vi "Serialize as XML.vi"(8 "error in (no error)":errorcluster, 10 "Nesting Level":i32, 11 "Attribute in":refnum<class "Attribute.lvclass">) -> (0 "error out":errorcluster, 2 "XML Fragment":string, 3 "Attribute out":refnum<class "Attribute.lvclass">)   [LabVIEW 2026, in "VILab.lvlib" / "Attribute.lvclass"]
uses:
  Attribute.lvclass
  Attribute.lvclass/Attribute.ctl
  Data Item/Data Item.lvclass
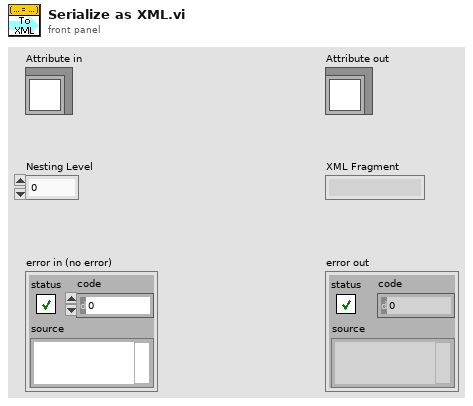
[diagram p1: front panel]
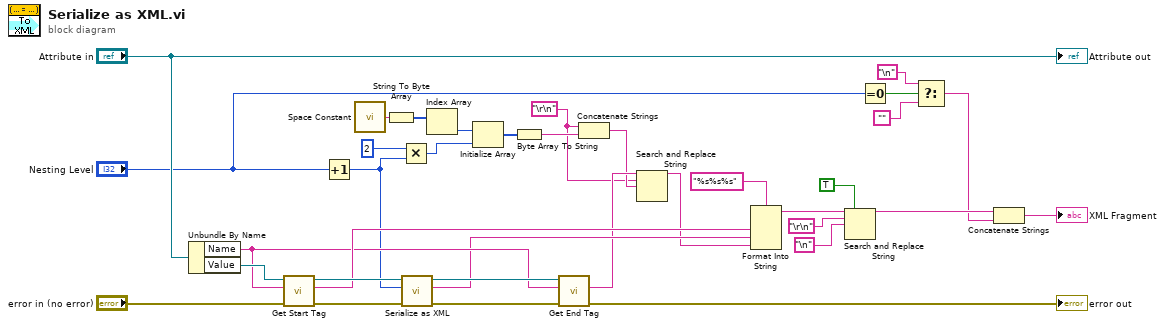
[diagram p0: block diagram]
diagram:
  w12 = "\r\n"
  n1 = Unbundle By Name("Attribute in") -> ("Name"=w25:string, "Value"=w28:refnum<class "Data Item.lvclass">)
  n2 = call-dynamic "Get Start Tag.vi"("error in (no error)"="error in (no error)", "Name"=w25, "Data Item in"=w28) -> ("error out"=w35:errorcluster, "Start Tag"=w26:string, "Data Item out"=w33:refnum<class "Data Item.lvclass">)  [unwired: 6 in]
  n3 = Increment(x="Nesting Level") -> (x+1=w13:i32)
  n4 = call <vilib>:"Space Constant.vi"() -> ("String"=w22:string)
  n5 = String To Byte Array(string=w22) -> (unsigned byte array=w21:u8[])
  n6 = Multiply(x=2 ("y"), y=w13) -> (x*y=w18:i32)
  n7 = call-dynamic "Serialize as XML.vi"("error in (no error)"=w35, "Nesting Level"=w13, "Data Item in"=w33) -> ("error out"=w31:errorcluster, "XML Fragment"=w24:string, "Data Item out"=w32:refnum<class "Data Item.lvclass">)  [unwired: 6 in]
  n8 = Index Array(array=w21) -> (element=w20:u8)  [unwired: 1 in]
  n9 = Initialize Array(w20, w18) -> (w19:u8[])
  n10 = Byte Array To String(unsigned byte array=w19) -> (string=w16:string)
  n11 = call-dynamic "Get End Tag.vi"("error in (no error)"=w31, "Name"=w25, "Data Item in"=w32) -> ("error out"=→"error out":errorcluster, "End Tag"=w17:string)  [unwired: 6 in, 1 out]
  n12 = Concatenate Strings(w12, w16) -> (w15:string)
  n13 = Search and Replace String(input string=w17, search string=w12, replace string=w15) -> (result string=w14:string)  [unwired: 5 in, 3 out]
  n14 = Format Into String(format string="%s%s%s", w26, w24, w14) -> (resulting string=w11:string)  [unwired: 2 in, 1 out]
  n15 = Search and Replace String(replace all?=TRUE ("replace all? (F)"), input string=w11, search string="\r\n", replace string="\n") -> (result string=w5:string)  [unwired: 4 in, 3 out]
  n16 = Equal To 0?(x="Nesting Level") -> (x = 0?=w6:bool)
  n17 = Select(t="\n", s=w6, f="") -> (s? t:f=w2:string)
  n18 = Concatenate Strings(w5, w2) -> (→"XML Fragment":string)
  "Attribute out" <- "Attribute in"
